vi "Read FPGA.vi"(0 "Refnum in":refnum<k20>, 1 "Front/Back Speed":u32, 2 "Front/Back in":enum16{"Forward", "Backward", "Stop"}(ring)=enum."Stop", 3 "Left/Right Speed":u32, 4 "Left/Right":enum16{"Left", "Right", "Stop"}(ring)=enum."Stop", 7 "error in (no error)":errorcluster, 8 "reference":refnum<vi>) -> (10 "Numeric 3":dbl, 12 "Front":dbl=37.140828371047974 format="%.2f", 15 "myRio / RC Control":bool, 16 "Front Side":dbl=39.974039793014526 format="%.2f", 17 "Right Radio":bool, 18 "myRio / RC Control 2":bool, 19 "State":T1(ring), 20 "Refnum out":refnum<k20>, 21 "Numeric 2":dbl, 22 "Left Radio":bool, 23 "Back Side":dbl=42.377978563308716 format="%.2f", 24 "Numeric":dbl, 25 "Back":dbl=166.97952270507812 format="%.2f", 26 "Time Elapsed":u32, 27 "error out":errorcluster)   [LabVIEW 2014]
uses:
  <vilib>/Utility/error.llb/Error Cluster From Error Code.vi
  <vilib>/rvi/errors/niLvFpgaAdjustHostInterfaceError.vi
  <vilib>/rvi/interface/nirviReadWriteControl/nirviReadWriteControl.xnode
  NiFpgaLv.dll
  <vilib>/rvi/interface/Simulation/niFpgaSimulationCallBeginRW.vi
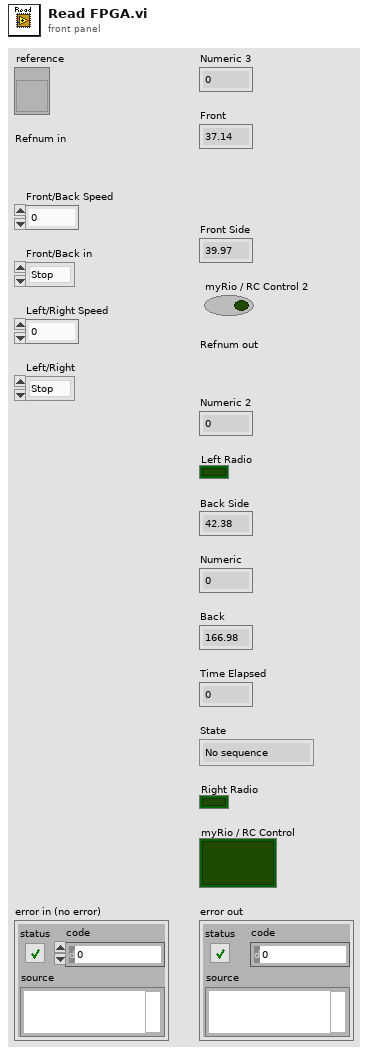
[diagram p1: front panel]
types:
  T1 = enum16{"No sequence", "Right 1", "Left 1", "Right 2", "Left 2"}
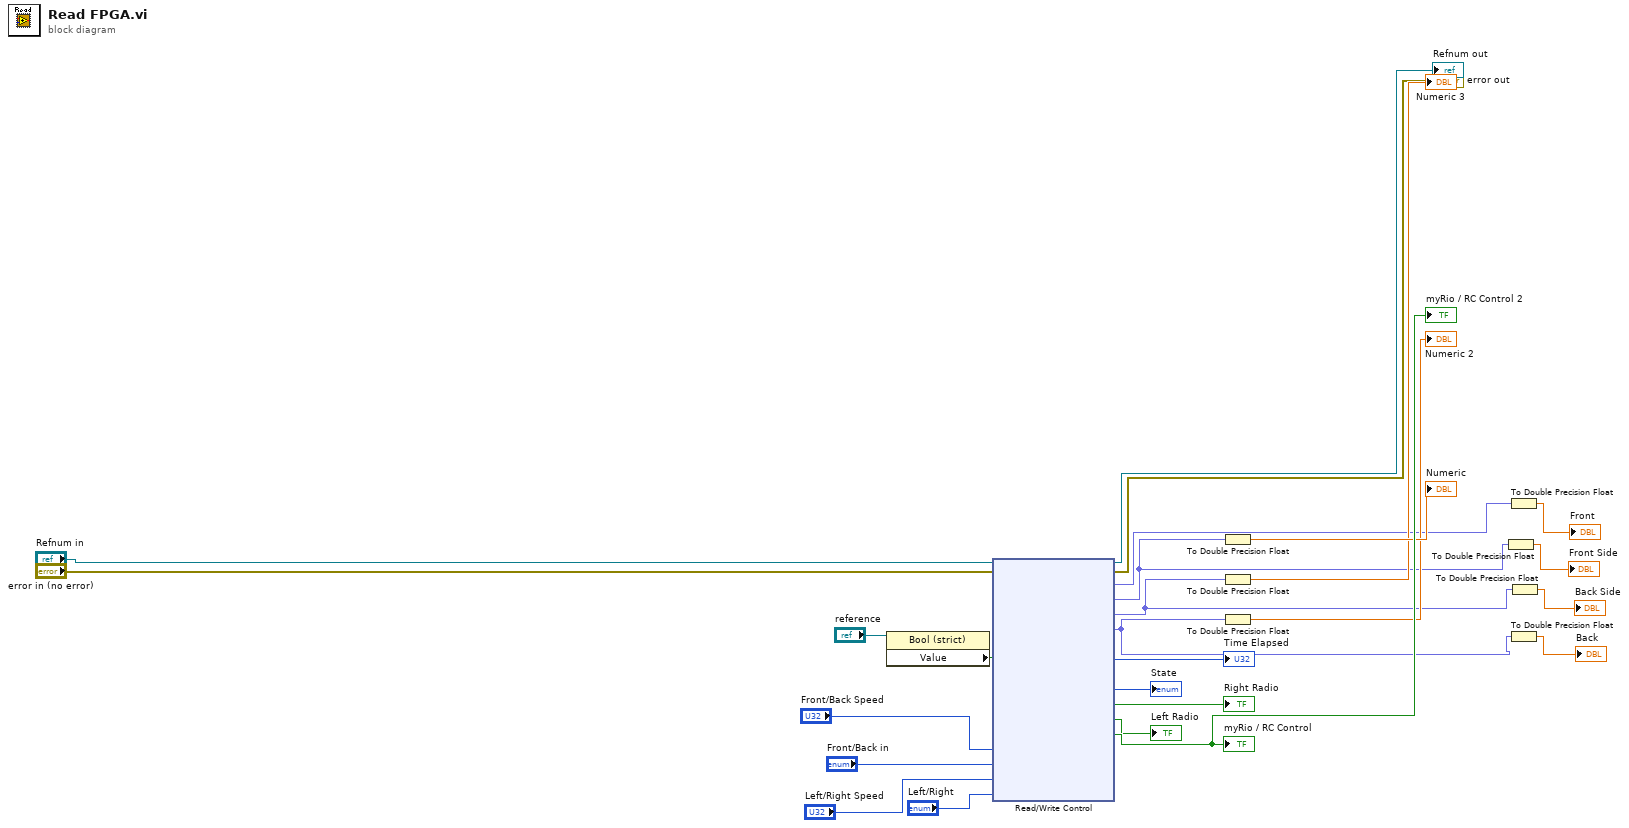
[diagram p0: block diagram]
diagram:
  n1 = property class="Bool (strict)"(reference="reference") -> ("Value"=w14:bool)  [unwired: 1 in, 2 out]
  n2 = xnode "Read/Write Control"("FPGA VI Reference In"="Refnum in", "error in"="error in (no error)", "STOP"=w14, "Front/Back Speed"="Front/Back Speed", "Front/Back 2"="Front/Back in", "Left/Right Speed"="Left/Right Speed", "Left/Right"="Left/Right") -> ("FPGA VI Reference Out"=→"Refnum out":refnum<k20>, "error out"=→"error out":errorcluster, "Front"=w8:fxp<+,64,16>, "Left"=w6:fxp<+,64,16>, "Right"=w4:fxp<+,64,16>, "Back"=w2:fxp<+,32,8>, "Time Elapsed"=→"Time Elapsed":u32, "State"=→"State":T1, "Right Radio"=→"Right Radio":bool, "Left Radio"=→"Left Radio":bool, "myRio / RC Control"=→"myRio / RC Control" →"myRio / RC Control 2":bool)  [unwired: 1 in]
  n3 = To Double Precision Float(number=w6) -> (double precision float=→"Numeric":dbl)
  n4 = To Double Precision Float(number=w4) -> (double precision float=→"Numeric 3":dbl)
  n5 = To Double Precision Float(number=w2) -> (double precision float=→"Numeric 2":dbl)
  n6 = To Double Precision Float(number=w6) -> (double precision float=→"Front Side":dbl)
  n7 = To Double Precision Float(number=w8) -> (double precision float=→"Front":dbl)
  n8 = To Double Precision Float(number=w2) -> (double precision float=→"Back":dbl)
  n9 = To Double Precision Float(number=w4) -> (double precision float=→"Back Side":dbl)
